vi "Append Block Diagram Image.vi"(0 "PDF Report IN":T25(xcontrol), 1 "Image size":T1={"Maximum Width"=-1, "Maximum Height"=-1}, 2 "Scale (%)":sgl=100.0, 3 "Border":T2={"Show?"=FALSE, "Thickness (point)"=0.5, "Color"=0}, 5 "VI reference":refnum<vi>, 11 "error in (no error)":errorcluster, 12 "Caption":string, 14 "Position and indentation":T3={"Alignment"=enum."Center", "X "=0.0, "Y"=0.0, "Indentation"=0.0}) -> (4 "PDF Report OUT":T25(xcontrol), 15 "error out":errorcluster)   [LabVIEW 2013]
doc: "Creates an image of the block diagram of the VI you specify in <B>VI reference</B> and appends it to a PDF report. <B>Not Available in Run-Time </B>.\n\n<B>FRANÇAIS</B>\nCréation de l'image du \"block diagram\" que vous avez spécifié par <B>VI reference</B> et ajout au rapport PDF. <B>Ce VI fonctionne uniquement en mode développement</B>.\n\nVersion 1.0\nDeveloped by Jean-Marc Simard\nCopyright © 2010, Exaprom Inc.\nAll rights reserved.\nLicense: BSD\n\nWith iTextSharp 4.1.6 (http://itextsharp.sourceforge.net)\nunder Mozilla Public License Version 1.1\n(http://www.mozilla.org/MPL/MPL-1.1.html)"
uses:
  Controls/PDF Report Xcontrol/PDF Report.xctl
  Controls/Image alignment and position.ctl
  Controls/Image aligment.ctl
  Controls/Image border.ctl
  Controls/Image Size Block Diagram.ctl
  Controls/Font cluster.ctl
  Controls/Font size.ctl
  Controls/Font color.ctl
  C:/Users/MaxCorp/Documents/GitHub/TopView/DLL/itextsharp.dll
  DLL/itextsharp.dll
panel:
  out "Size (points)":cluster{"TotalHeight":sgl, "TotalWidth":sgl}
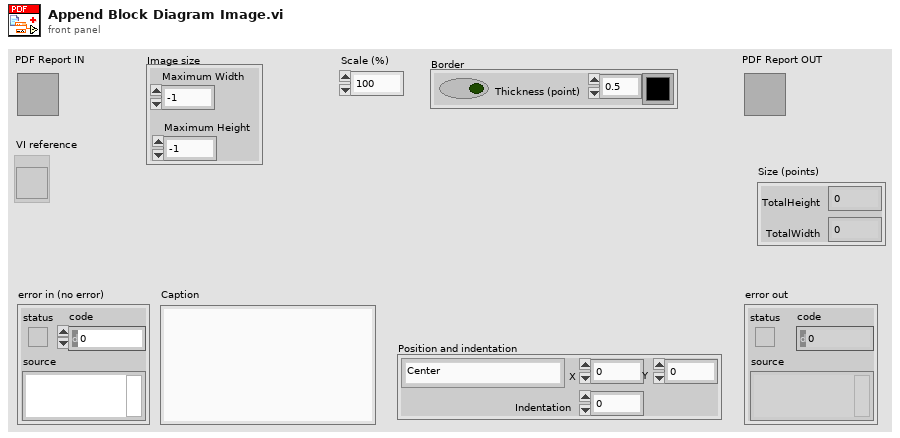
[diagram p1: front panel]
types:
  T1 = typedef "Image Size Block Diagram.ctl" = cluster{"Maximum Width":i32, "Maximum Height":i32}
  T2 = typedef "Image border.ctl" = cluster{"Show?":bool, "Thickness (point)":sgl, "Color":u32}
  T3 = typedef "Image alignment and position.ctl" = cluster{"Alignment":T4, "X ":sgl, "Y":sgl, "Indentation":sgl}
  T4 = typedef "Image aligment.ctl" = enum16{"Absolute (X,Y) in mm", "Left", "Center", "Right", "Left (textwrap)", "Right (textwrap)"}
  T5 = typedef "Font cluster.ctl" = cluster{"Name":string, "Size":T6, "Color":T7, "Style":cluster{"Bold":bool, "Italic":bool, "Underline":bool, "Strikeout":bool}}
  T6 = typedef "Font size.ctl" = sgl
  T7 = typedef "Font color.ctl" = u32
  T8 = typedef "Unit.ctl" = enum16{"inch", "mm"}
  T9 = typedef "Paragraphe cluster.ctl" = cluster{" Aligment":T10, "Line spacing":T11}
  T10 = typedef "Texte alignement.ctl" = enum16{"Select", "CENTER", "JUSTIFY", "LEFT", "RIGHT"}
  T11 = typedef "Line spacing.ctl" = enum16{"Select", "1.0", "1.5", "2.0"}
  T12 = typedef "Page dimensions.ctl" = cluster{"Start at page":i32, "Orientation":T13, "widht":sgl, "height":sgl, "Margin left":sgl, "Margin right":sgl, "Margin top":sgl, "Margin bottom":sgl}
  T13 = typedef "Page Orientation.ctl" = enum16{"Portrait", "Landscape"}
  T14 = typedef "Image or Table Caption.ctl" = cluster{"Caption":string, "Separator":string, "Position":enum16{"Above", "Below"}}
  T15 = typedef "Header Footer [ ].ctl" = T16[]
  T16 = typedef "Header Footer cluster.ctl" = cluster{"Start page":i32, "Type":T17, "Alignment":T18, "Vertical Alignement":T19, "Image (%)":sgl, "Page #":T20, "Text":string, "Path":string, "Font":T5, "Font refnum":refnum<k24>, "Line":cluster{"Line":T21, "Thickness (points)":sgl, "Colour":T7}}
  T17 = typedef "Header Footer Type.ctl" = enum16{"Select", "Text", "Text + hyperlink", "Page number", "Image", "Image + hyperlink"}
  T18 = typedef "Header footer horiz alignment.ctl" = enum16{"Left", "Center", "Right"}
  T19 = typedef "Cell Vertical alignment.ctl" = enum16{"TOP", "MIDDLE", "BOTTOM"}
  T20 = typedef "Page number.ctl" = cluster{"Text 1":string, "Text 2":string, "Text 3":string}
  T21 = typedef "Header Footer Line.ctl" = enum16{"No line", "Horizontal line"}
  T22 = typedef "Watermark cluster2.ctl" = cluster{"Show? (F)":bool, "Type":enum16{"Image", "Text"}, "Opacity (%)":sgl, "Rotate(°)":sgl, "Position":cluster{"Position":T23, "X":sgl, "Y":sgl}, "Image path":path, "Scaled(%)":sgl, "Image refnum":refnum<k24>, "Text":string, "Font":cluster{"Name":string, "Size":T6, "Color":T7}, "Font refnum":refnum<k24>, "Alignment":T18, "Automatic":bool}
  T23 = typedef "Watermark Position.ctl" = enum16{"Absolute", "Center (page)", "Center (text section)"}
  T24 = typedef "System Fonts.ctl" = cluster{"Font name [ ]":string[], "Font and file names [ ]":cluster{"Font name":string, "File name":string}[]}
  T25 = cluster{"Document":refnum<k24>, "Writer":refnum<k24>, "Default Font":refnum<k24>, "Default Font cluster":T5, "Path":path, "Unit (default = mm)":T8, "Paragraphe cluster":T9, "Pages dimensions [ ]":T12[], "Captions":cluster{"Image":T14, "Image counter":u16, "Table":T14, "Table counter":u16, "Font":T5}, "Header":T15, "Footer":T15, "Watermark ":T22, "Actual VI name":string, "System Fonts":T24}
  T26 = enum32{"invalid app kind", "Development System", "Run Time System", "Student Edition", "Embedded LabVIEW", "Evaluation", "Custom"}
  T27 = typedef "imagedata.ctl" = cluster{"image type":i32, "image depth":i32, "image":u8[], "mask":u8[], "colors":u32[], "Rectangle":cluster{"left":i16, "top":i16, "right":i16, "bottom":i16}}
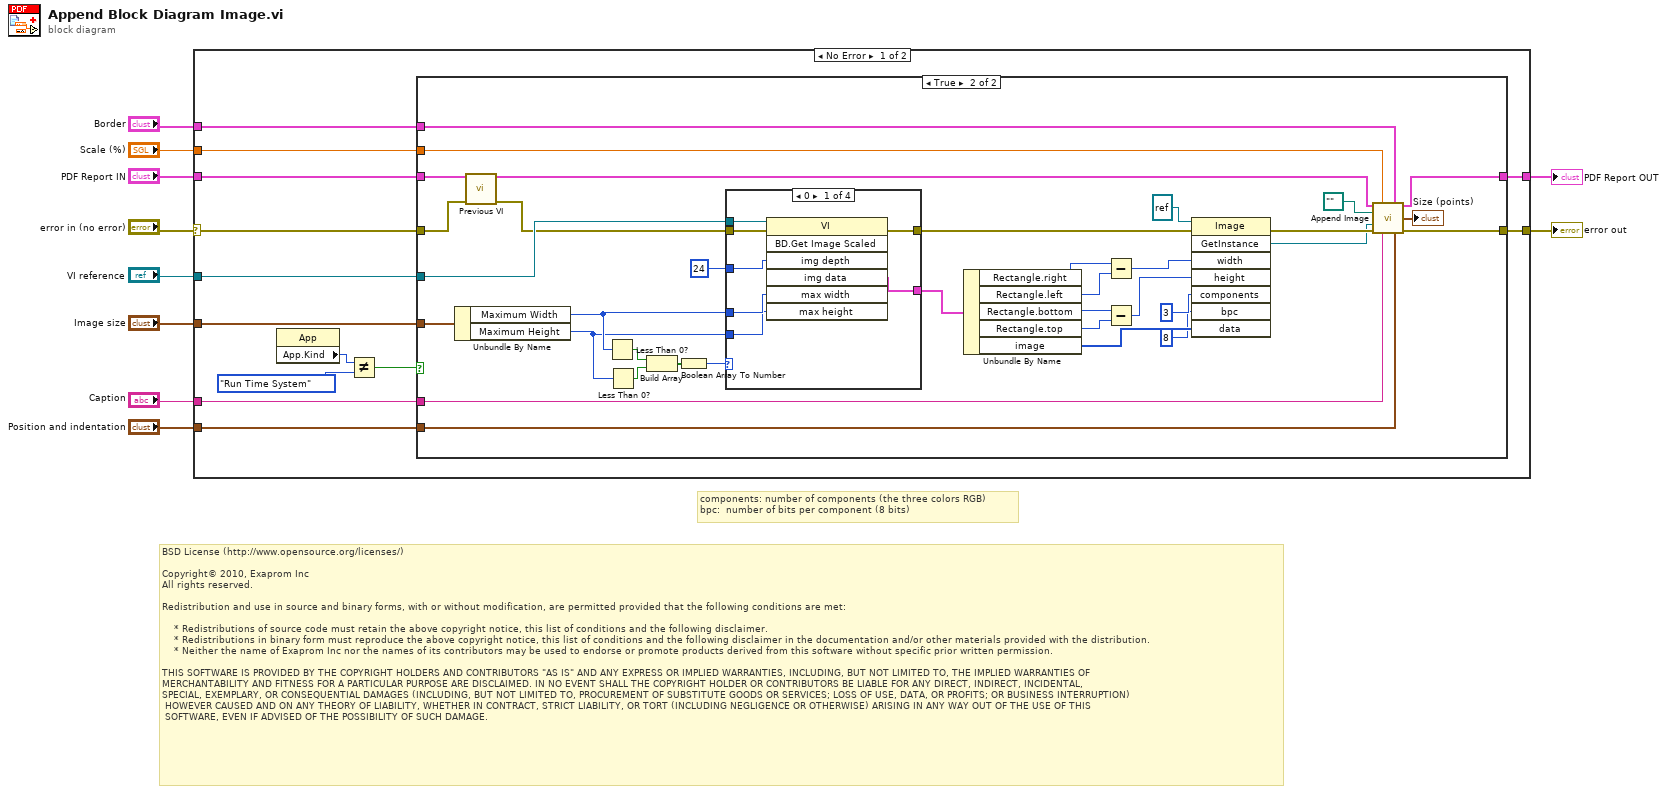
[diagram p0: block diagram]
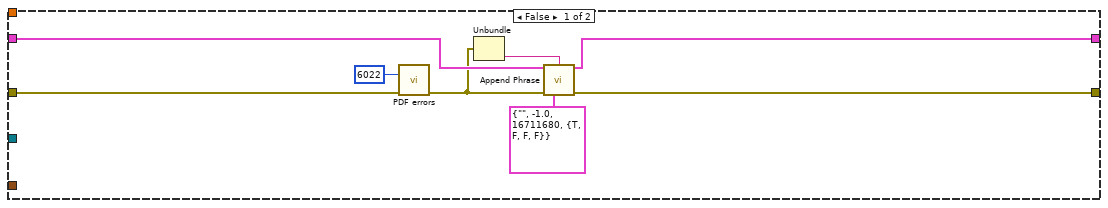
[diagram p2: hidden frame]
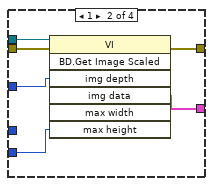
[diagram p3: hidden frame]
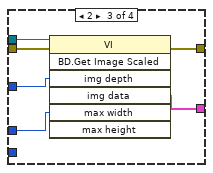
[diagram p4: hidden frame]
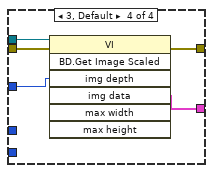
[diagram p5: hidden frame]
diagram:
  # "components: number of components (the three colors RGB)\nbpc:  number of bits per component (8 bits)"
  # "BSD License (http://www.opensource.org/licenses/)\n\nCopyright© 2010, Exaprom Inc\nAll rights reserved.\n\nRedistribution and use in source and binary forms, with or without modification, are permitted provided that the following conditions are met:\n\n    * Redistributions of source code must retain the above copyright notice, this list of conditions and the following disclaimer.\n    * Redistributions in binary form must reproduce the above copyright notice, this list of conditions and the following disclaimer in the documentation and/or other materials provided with the distribution.\n    * Neither the name of Exaprom Inc nor the names of its contributors may be used to endorse or promote products derived from this software without specific prior written permission.\n\nTHIS SOFTWARE IS PROVIDED BY THE COPYRIGHT HOLDERS AND CONTRIBUTORS \"AS IS\" AND ANY EXPRESS OR IMPLIED WARRANTIES, INCLUDING, BUT NOT LIMITED TO, THE IMPLIED WARRANTIES OF \nMERCHANTABILITY AND FITNESS FOR A PARTICULAR PURPOSE ARE DISCLAIMED. IN NO EVENT SHALL THE COPYRIGHT HOLDER OR CONTRIBUTORS BE LIABLE FOR ANY DIRECT, INDIRECT, INCIDENTAL,\nSPECIAL, EXEMPLARY, OR CONSEQUENTIAL DAMAGES (INCLUDING, BUT NOT LIMITED TO, PROCUREMENT OF SUBSTITUTE GOODS OR SERVICES; LOSS OF USE, DATA, OR PROFITS; OR BUSINESS INTERRUPTION)\n HOWEVER CAUSED AND ON ANY THEORY OF LIABILITY, WHETHER IN CONTRACT, STRICT LIABILITY, OR TORT (INCLUDING NEGLIGENCE OR OTHERWISE) ARISING IN ANY WAY OUT OF THE USE OF THIS\n SOFTWARE, EVEN IF ADVISED OF THE POSSIBILITY OF SUCH DAMAGE."
  n1 = case shown="No Error" "error in (no error)" {
    selector: "error in (no error)" -> [w15 w92]
    tunnel: [w20 w92] -> w3
    tunnel: "VI reference" -> [w23 _]
    tunnel: [w21 w91] -> w2
    tunnel: "PDF Report IN" -> [w22 w91]
    tunnel: "Caption" -> [w19 _]
    tunnel: "Position and indentation" -> [w18 _]
    tunnel: "Border" -> [w17 _]
    tunnel: "Scale (%)" -> [w16 _]
    tunnel: "Image size" -> [w14 _]
    frame No Error {
      n2 = property class="App"() -> ("App.Kind"=w12:T26)  [unwired: 2 in, 2 out]
      n3 = Not Equal?(x=w12, y=T26."Run Time System") -> (x != y?=w11:bool)
      n4 = case shown="True" w11 {
        tunnel: w23 -> [_ w66]
        tunnel: w22 -> [w29 w63]
        tunnel: [w28 w62] -> w21
        tunnel: [w27 w61] -> w20
        tunnel: w19 -> [_ w60]
        tunnel: w18 -> [_ w59]
        tunnel: w17 -> [_ w58]
        tunnel: w16 -> [_ w57]
        tunnel: w15 -> [w31 w54]
        tunnel: w14 -> [_ w52]
        frame False {
          n5 = call "PDF errors.vi"("code"=6022, "error in (no error)"=w31) -> ("error out"=w26:errorcluster)  [unwired: 1 in, 12 out]
          n6 = Unbundle(w26) -> ("source"=w25:string)  [unwired: 2 out]
          n7 = call "Append Phrase.vi"("PDF Report IN"=w29, "Text"=w25, "error in (no error)"=w26, "Font"=T5 {"Name"="", "Size"=-1.0, "Color"=16711680, "Style"={"Bold"=TRUE, "Italic"=FALSE, "Underline"=FALSE, "Strikeout"=FALSE}}) -> ("PDF Report OUT"=w28:T25, "error out"=w27:errorcluster)  [unwired: 1 in, 9 out]
        }
        frame True {
          n8 = Unbundle By Name(w52) -> ("Maximum Width"=w37:i32, "Maximum Height"=w36:i32)
          n9 = call "Previous VI.vi"("PDF Report IN"=w63, "error in (no error)"=w54) -> ("PDF Report OUT"=w51:T25, "error out"=w53:errorcluster)  [unwired: 12 out]
          n10 = Less Than 0?(x=w37) -> (x < 0?=w35:bool)
          n11 = Less Than 0?(x=w36) -> (x < 0?=w34:bool)
          n12 = Build Array(w35, w34) -> (w33:bool[])
          n13 = Boolean Array To Number(Boolean array=w33) -> (number=w32:u32)
          n14 = case shown="0" w32 {
            tunnel: [w73 w79 w85 w90] -> w50
            tunnel: w66 -> [w72 w78 w84 w89]
            tunnel: [w71 w77 w83 w88] -> w39
            tunnel: 24 ("Image Depth") -> [w70 w76 w82 w87]
            tunnel: w53 -> [w69 w75 w81 w86]
            tunnel: w37 -> [w68 _ w80 _]
            tunnel: w36 -> [w67 w74 _ _]
            frame 0 {
              n15 = invoke class="VI" method="BD.Get Image Scaled"(reference=w72, error in=w69, "img depth"=w70, "max width"=w68, "max height"=w67) -> (error out=w73:errorcluster, "img data"=w71:T27)  [unwired: 2 in, 5 out]
            }
            frame 1 {
              n16 = invoke class="VI" method="BD.Get Image Scaled"(reference=w78, error in=w75, "img depth"=w76, "max height"=w74) -> (error out=w79:errorcluster, "img data"=w77:T27)  [unwired: 3 in, 5 out]
            }
            frame 2 {
              n17 = invoke class="VI" method="BD.Get Image Scaled"(reference=w84, error in=w81, "img depth"=w82, "max width"=w80) -> (error out=w85:errorcluster, "img data"=w83:T27)  [unwired: 3 in, 5 out]
            }
            frame 3, Default {
              n18 = invoke class="VI" method="BD.Get Image Scaled"(reference=w89, error in=w86, "img depth"=w87) -> (error out=w90:errorcluster, "img data"=w88:T27)  [unwired: 4 in, 5 out]
            }
          }
          n19 = Unbundle By Name(w39) -> ("Rectangle.right"=w48:i16, "Rectangle.left"=w47:i16, "Rectangle.bottom"=w45:i16, "Rectangle.top"=w44:i16, "image"=w41:u8[])
          n20 = Subtract(x=w48, y=w47) -> (x-y=w46:i16)
          n21 = Subtract(x=w45, y=w44) -> (x-y=w43:i16)
          n22 = invoke class="Image" method="GetInstance"(reference=refnum<k24> refnum ("image"), error in=w50, "width"=w46, "height"=w43, "components"=3, "bpc"=8, "data"=w41) -> (error out=w64:errorcluster, "GetInstance"=w56:refnum<k24>)  [unwired: 1 in, 6 out]
          n23 = call "Append Image.vi"("PDF Report IN"=w51, "Scale (%)"=w57, "Border"=w58, "Image path"=path "" ("path"), "Image Ref iTexSharp"=w56, "error in (no error)"=w64, "Caption"=w60, "Position and indentation"=w59) -> ("PDF Report OUT"=w62:T25, "Size (points)"=→"Size (points)":cluster{"TotalHeight":sgl, "TotalWidth":sgl}, "error out"=w61:errorcluster)  [unwired: 5 out]
        }
      }
    }
    frame Error {
    }
  }
  "error out" <- w3
  "PDF Report OUT" <- w2
